vi "programa 8.vi"() -> ()   [LabVIEW 2012]
panel:
  out "Array 2":dbl[](array[numeric])
  out "SumaColumna":dbl
  in  "Columna":dbl
  out "SumaLinea":dbl
  in  "Linea":dbl
  out "Array":dbl[][](array[numeric])
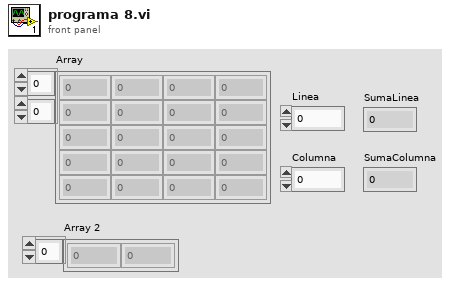
[diagram p1: front panel]
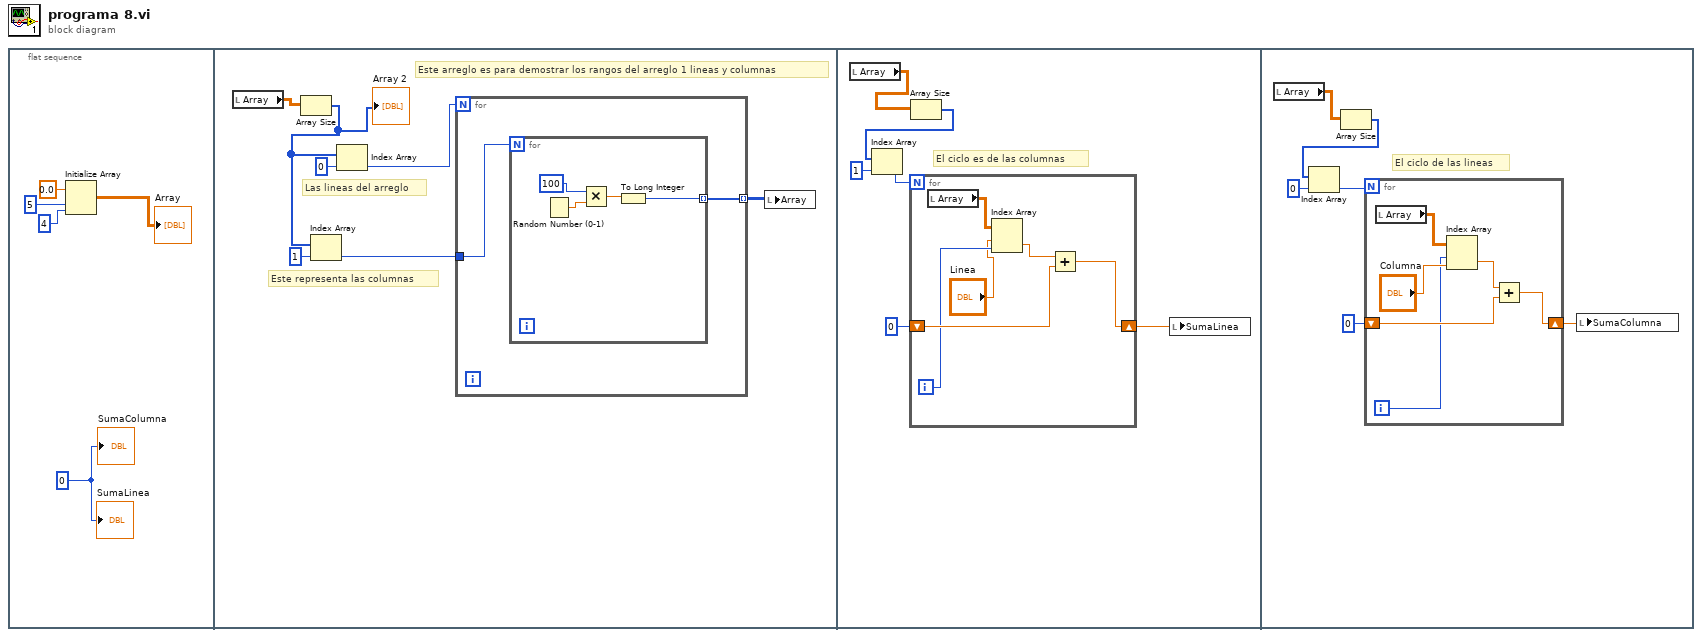
[diagram p0: block diagram]
diagram:
  n1 = flat-sequence {
    frame #0 {
      w1 = 0
      n2 = Initialize Array "Initialize Array"(0.0 ("element"), 5, 4) -> (→"Array":dbl[][])
      "SumaColumna" <- w1
      "SumaLinea" <- w1
    }
    frame #1 {
      # "Este arreglo es para demostrar los rangos del arreglo 1 lineas y columnas"
      # "Este representa las columnas"
      # "Las lineas del arreglo"
      n3 = local read "Array"() -> (w11:dbl[][])
      n4 = Array Size(array=w11) -> (size(s)=w6:i32[])
      "Array 2" <- w6
      n5 = Index Array(array=w6, index=1) -> (element=w7:i32)
      n6 = Index Array "Index Array"(array=w6, index=0) -> (element=w8:i32)
      n7 = for {
        N: w8 -> [_]
        tunnel: [w14] -> w12 mode=indexing
        tunnel: w7 -> [w13]
        n8 = for {
          N: w13 -> [_]
          tunnel: [w15] -> w14 mode=indexing
          n9 = Random Number (0-1)() -> (number: 0 to 1=w17:dbl)
          n10 = Multiply(x=100, y=w17) -> (x*y=w16:dbl)
          n11 = To Long Integer(number=w16) -> (32bit integer=w15:i32)
        }
      }
      n12 = local write "Array"(w12) -> ()
    }
    frame #2 {
      # "El ciclo es de las columnas"
      n13 = local read "Array"() -> (w24:dbl[][])
      n14 = Array Size(array=w24) -> (size(s)=w19:i32[])
      n15 = Index Array "Index Array"(array=w19, index=1) -> (element=w22:i32)
      n16 = for {
        N: w22 -> [_]
        shift-right: [w25] -> w20
        shift-left: 0 -> [w28]
        i -> [w27]
        n17 = local read "Array"() -> (w30:dbl[][])
        n18 = Index Array "Index Array"(array=w30, index (row)="Linea", index (col)=w27) -> (element=w29:dbl)
        n19 = Add(x=w29, y=w28) -> (x+y=w25:dbl)
      }
      n20 = local write "SumaLinea"(w20) -> ()
    }
    frame #3 {
      # "El ciclo de las lineas"
      n21 = local read "Array"() -> (w36:dbl[][])
      n22 = Array Size(array=w36) -> (size(s)=w35:i32[])
      n23 = Index Array "Index Array"(array=w35, index=0) -> (element=w33:i32)
      n24 = for {
        N: w33 -> [_]
        shift-right: [w39] -> w31
        shift-left: 0 -> [w40]
        i -> [w37]
        n25 = local read "Array"() -> (w42:dbl[][])
        n26 = Index Array "Index Array"(array=w42, index (row)=w37, index (col)="Columna") -> (element=w41:dbl)
        n27 = Add(x=w41, y=w40) -> (x+y=w39:dbl)
      }
      n28 = local write "SumaColumna"(w31) -> ()
    }
  }
